vi "arduinotalker.vi"() -> ()   [LabVIEW 2021]
uses:
  <vilib>/Instr/_visa.llb/VISA Configure Serial Port (Instr).vi
panel:
  in  "Boolean":bool
  in  "VISA resource name":refnum<visa-resource-name>
  in  "stop":bool
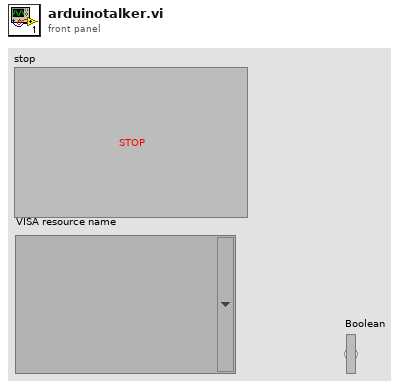
[diagram p1: front panel]
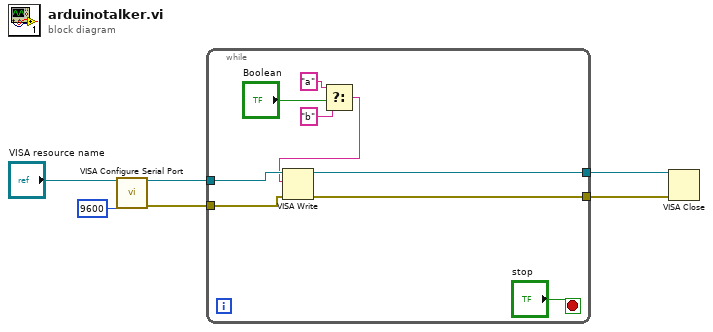
[diagram p0: block diagram]
diagram:
  n1 = call-poly "VISA Configure Serial Port"("VISA resource name"="VISA resource name", "baud rate (9600)"=u32 9600) -> ("VISA resource name out"=w4:refnum<visa-resource-name>, "error out"=w2:errorcluster)  [unwired: 12 in]
  n2 = while {
    tunnel: w4 -> [w14]
    tunnel: [w13] -> w3
    tunnel: w2 -> [w12]
    tunnel: [w11] -> w1
    stop <- "stop" stop-if-true
    n3 = Select(t="a", s="Boolean", f="b") -> (s? t:f=w7:string)
    n4 = VISA Write(VISA resource name=w14, write buffer=w7, error in (no error)=w12) -> (VISA resource name out=w13:refnum<visa-resource-name>, error out=w11:errorcluster)  [unwired: 1 out]
  }
  n5 = VISA Close(VISA resource name=w3, error in (no error)=w1) -> ()  [unwired: 1 out]
